vi "Test - Serial Device - Read ADC 1.vi"(8 "error in (no error)":errorcluster, 11 "Module ID":i32) -> (0 "error out":errorcluster, 3 "Pass":bool)   [LabVIEW 2020]
doc: "_____\nCreated using Delacor QMH Event Scripter 5.0.0.112."
uses:
  Libraries/Serial Device/Serial Device.lvlib
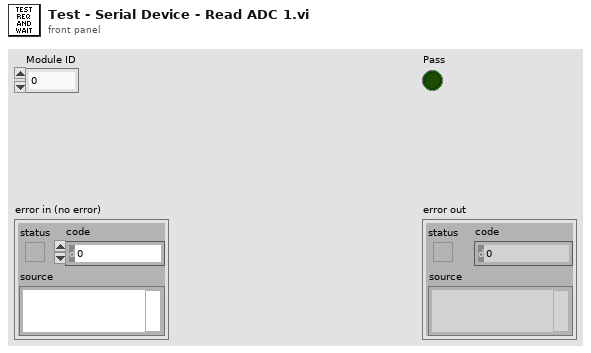
[diagram p1: front panel]
types:
  T1 = typedef "Serial Device.lvlib/Read ADC (Reply Payload)--cluster.ctl" = cluster{"Read ADC_error":errorcluster, "Response":string}
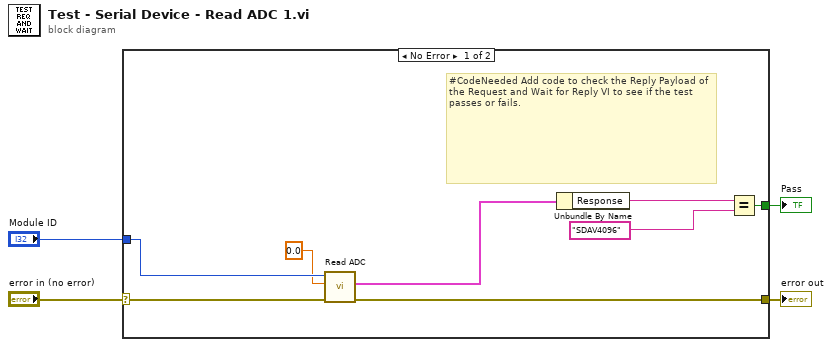
[diagram p0: block diagram]
diagram:
  n1 = case shown="No Error" "error in (no error)" {
    selector: "error in (no error)" -> [w12 w13]
    tunnel: [w11 w13] -> w3
    tunnel: "Module ID" -> [w10 _]
    tunnel: [w9 _] -> w1
    frame No Error {
      # "#CodeNeeded Add code to check the Reply Payload of the Request and Wait for Reply VI to see if the test passes or fails."
      n2 = call "Read ADC.vi"("error in (no error)"=w12, "Channel"=0.0, "Module ID"=w10) -> ("error out"=w11:errorcluster, "Reply Payload"=w8:T1)  [unwired: 6 in, 1 out]
      n3 = Unbundle By Name(w8) -> ("Response"=w7:string)
      n4 = Equal?(x=w7, y="SDAV4096" ("Respuestas")) -> (x = y?=w9:bool)
    }
    frame Error {
    }
  }
  "error out" <- w3
  "Pass" <- w1
